vi "i2clib_read.vi"(8 "error in (no error)":errorcluster, 9 "recv_size":i32, 10 "dev_addr":u8, 11 "I2C Reference":i32) -> (0 "error out":errorcluster, 2 "recv_data":u8[](array[numeric]), 3 "I2C Reference Out":i32)   [LabVIEW 2017]
uses:
  <vilib>/Utility/error.llb/Error Cluster From Error Code.vi
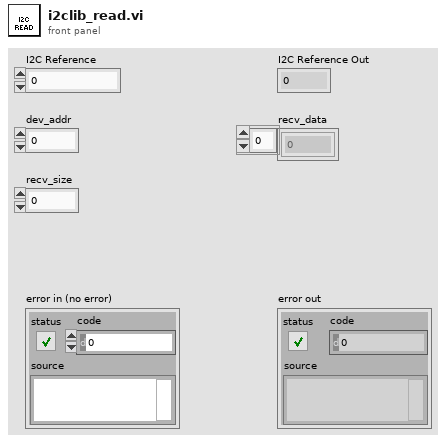
[diagram p1: front panel]
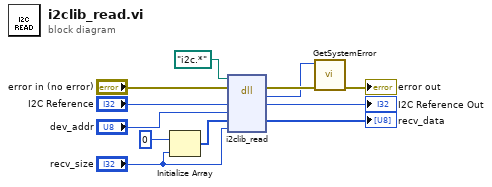
[diagram p0: block diagram]
diagram:
  n1 = Initialize Array(i8 0 ("dev_addr"), "recv_size") -> (w6:i8[])
  n2 = dll-call lib="?" fn="i2clib_read"(path in=path "i2c.*", error in="error in (no error)", "handle"="I2C Reference", "dev_addr"="dev_addr", "recv_buf"=w6, "recv_size"="recv_size") -> (error out=w4:errorcluster, "return type"=w2:i32, "handle"=→"I2C Reference Out":i32, "recv_buf"=→"recv_data":i8[])  [unwired: 3 in, 1 out]
  n3 = call <vilib>:"GetSystemError.vi"("error in (no error)"=w4, "Retval"=w2) -> ("error out"=→"error out":errorcluster)  [unwired: 9 in]
